vi "Mask Write Holding Register.vi"(4 "OR mask":u16, 6 "AND mask":u16, 8 "error in (no error)":errorcluster, 10 "address":u16, 11 "device data model in":refnum<class "Device Data Model.lvclass">) -> (0 "error out":errorcluster, 3 "device data model out":refnum<class "Device Data Model.lvclass">)   [LabVIEW 2020, in "SubVIs.lvlib" / "Device Data Model.lvclass"]
doc: "Writes the masked value of a single register using an <b>AND mask</b> and an <b>OR mask</b> using the equation below:\nResult=(Current Value AND AndMask) OR (OrMask AND !AndMask)"
uses:
  <vilib>/Modbus/subvis/Data and Functions/Device Data Model/Device Data Model.lvclass
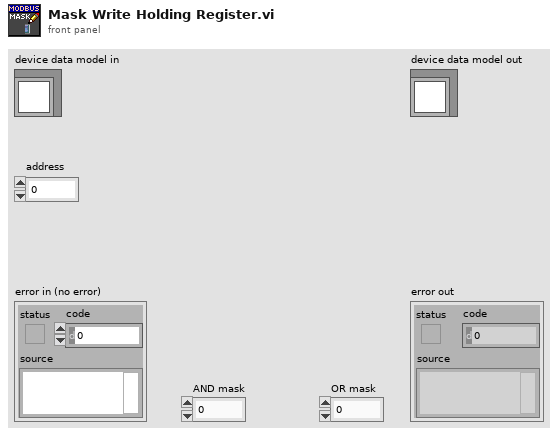
[diagram p1: front panel]
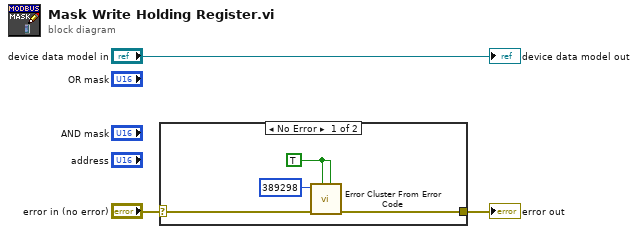
[diagram p0: block diagram]
diagram:
  n1 = case shown="No Error" "error in (no error)" {
    selector: "error in (no error)" -> [w7 w8]
    tunnel: [w6 w8] -> w1
    frame No Error {
      w4 = TRUE ("show call chain? (False)")
      n2 = call <vilib>:"Error Cluster From Error Code.vi"("is warning? (False)"=w4, "show call chain? (False)"=w4, "error in (no error)"=w7, "error code (0)"=389298) -> ("error out"=w6:errorcluster)  [unwired: 5 in]
    }
    frame Error {
    }
  }
  "error out" <- w1
  "device data model out" <- "device data model in"
